vi "TSCANFD_SetData.vi"(8 "错误输入（无错误）":errorcluster, 10 "CANFD配置":T1={"硬件类型"=8, "硬件子类型"=0, "AArbRateKbps"=250.0, "AListenOnly"=enum."Normal", "Int120Ohm"=enum."Enable", "EnableChannel"=enum."Enable", "AHwChannel"=0, "AAppChannel"=0, "ADataRateKbps"=250.0, "AControllerType"=0, "AControllerMode"=0} {"硬件类型" items=["BUS_UNKNOWN_TYPE", "TS_TCP_DEVICE", "XL_USB_DEVICE", "TS_USB_DEVICE", "PEAK_USB_DEVICE", "KVASER_USB_DEVICE", "ZLG_USB_DEVICE", "ICS_USB_DEVICE", "TS_TC1005_DEVICE"]; "硬件子类型" items=["BUS_UNKNOWN_TYPE", "TSCAN_PRO_4", "TSCAN_LITE_2", "TSCANMini", "TSLinMini", "TSCANFDmini", "TSCAN_LIN_IO_2", "TSCAN_LITE_2", "TSCANLIN", "TSCAN_FD_Mini_1"]; "AHwChannel" items=["CHN1", "CHN2", "CHN3", "CHN4", "CHN5", "CHN6", "CHN7", "CHN8", "CHN9", "CHN10", "CHN11", "CHN12", "CHN13", "CHN14", "CHN15", "CHN16", "CHN17", "CHN18", "CHN19", "CHN20", "CHN21", "CHN22", "CHN23", "CHN24", "CHN25", "CHN26", "CHN27", "CHN28", "CHN29", "CHN30", "CHN31", "CHN32"]; "AAppChannel" items=["CHN1", "CHN2", "CHN3", "CHN4", "CHN5", "CHN6", "CHN7", "CHN8", "CHN9", "CHN10", "CHN11", "CHN12", "CHN13", "CHN14", "CHN15", "CHN16", "CHN17", "CHN18", "CHN19", "CHN20", "CHN21", "CHN22", "CHN23", "CHN24", "CHN25", "CHN26", "CHN27", "CHN28", "CHN29", "CHN30", "CHN31", "CHN32"]; "AControllerType" items=["lfdtCAN", "lfdtISOFDCAN", "lfdtNonISOFDFDCAN"]; "AControllerMode" items=["lfdmNormal", "lfdmACKOff", "lfdmRestricted"]}, 11 "路径输入":path) -> (0 "错误输出":errorcluster, 2 "AAPPChannel":i32, 3 "路径输出":path, 4 "Set_Baudrated_Successfully":bool, 6 "Mapping_Successfully":bool)   [LabVIEW 2019]
panel:
  # "用N路can通道，设置N路CAN通道"
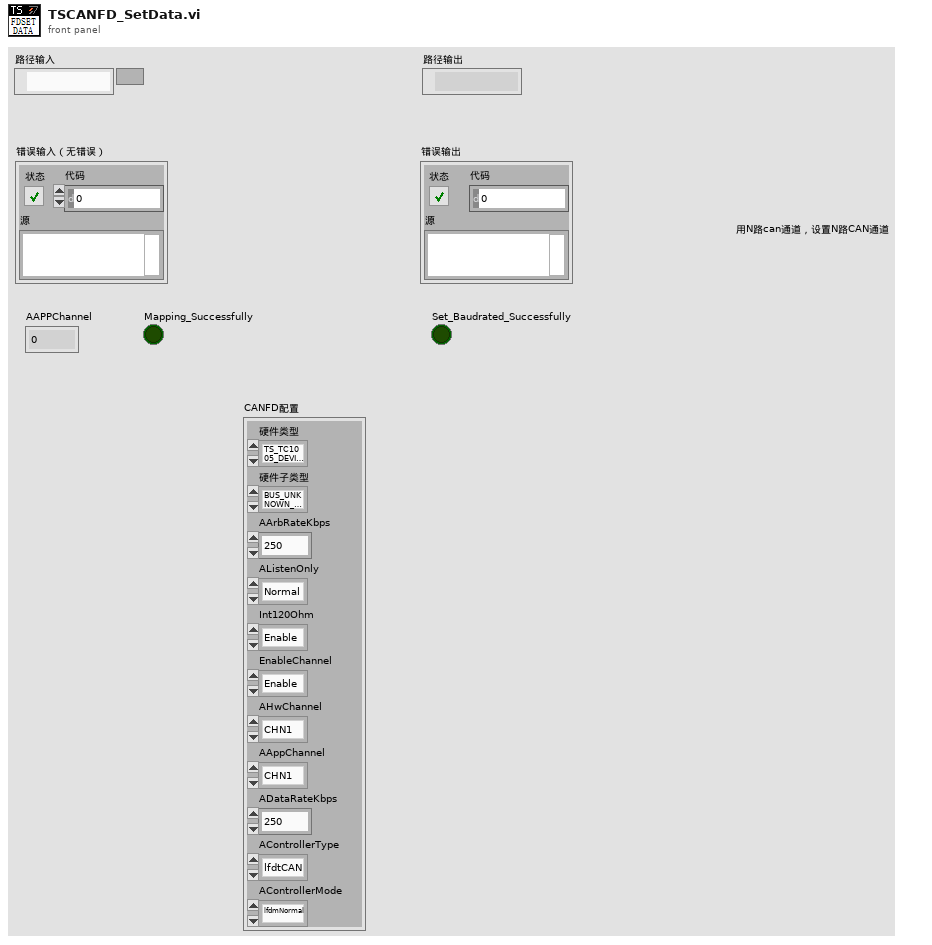
[diagram p1: front panel]
types:
  T1 = cluster{"硬件类型":i32, "硬件子类型":i32, "AArbRateKbps":sgl, "AListenOnly":enum16{"Normal", "ListenOnly"}, "Int120Ohm":enum16{"Disable", "Enable"}, "EnableChannel":enum16{"Disable", "Enable"}, "AHwChannel":i32, "AAppChannel":i32, "ADataRateKbps":sgl, "AControllerType":i32, "AControllerMode":i32}
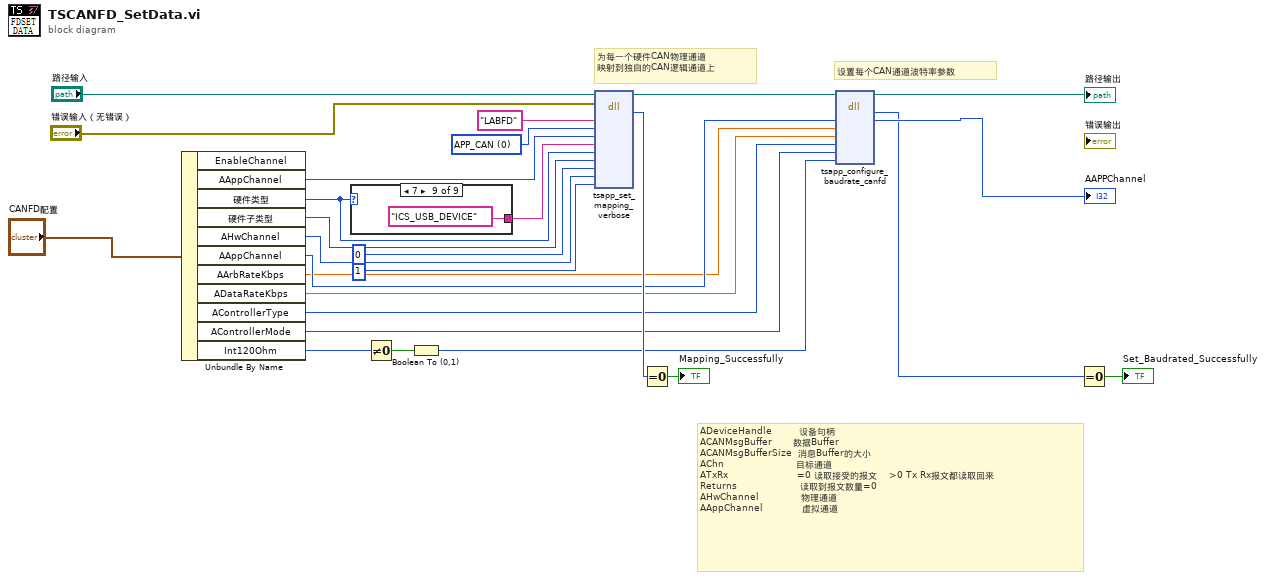
[diagram p0: block diagram]
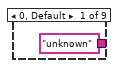
[diagram p2: hidden frame]
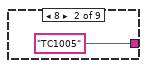
[diagram p3: hidden frame]
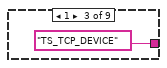
[diagram p4: hidden frame]
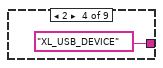
[diagram p5: hidden frame]
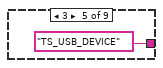
[diagram p6: hidden frame]
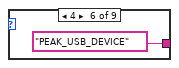
[diagram p7: hidden frame]
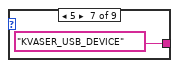
[diagram p8: hidden frame]
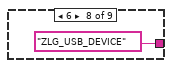
[diagram p9: hidden frame]
diagram:
  w26 = 0 items=["APP_CAN", "APP_LIN"] ("AAppChannelType")
  # "ADeviceHandle         设备句柄\nACANMsgBuffer       数据Buffer\nACANMsgBufferSize  消息Buffer的大小\nAChn                        目标通道\nATxRx                       =0 读取接受的报文    >0 Tx Rx报文都读取回来\nReturns                     读取到报文数量=0\nAHwChannel              物理通道\nAAppChannel             虚拟通道"
  # "设置每个CAN通道波特率参数"
  # "为每一个硬件CAN物理通道\n映射到独自的CAN逻辑通道上"
  n1 = Unbundle By Name("CANFD配置") -> ("AAppChannel"=w25:i32, "硬件类型"=w23:i32, "硬件子类型"=w22:i32, "AHwChannel"=w20:i32, "AAppChannel"=w9:i32, "AArbRateKbps"=w7:sgl, "ADataRateKbps"=w6:sgl, "AControllerType"=w5:i32, "AControllerMode"=w4:i32, "Int120Ohm"=w17:enum16{"Disable", "Enable"})  [unwired: 1 out]
  n2 = case shown="7" w23 {
    tunnel: ["unknown" ("AHardwareName") "TC1005" ("AHardwareName") "TS_TCP_DEVICE" ("AHardwareName") "XL_USB_DEVICE" ("AHardwareName") "TS_USB_DEVICE" ("AHardwareName") "PEAK_USB_DEVICE" ("AHardwareName") "KVASER_USB_DEVICE" ("AHardwareName") "ZLG_USB_DEVICE" ("AHardwareName") "ICS_USB_DEVICE" ("AHardwareName")] -> w24
    frame 0, Default {
    }
    frame 8 {
    }
    frame 1 {
    }
    frame 2 {
    }
    frame 3 {
    }
    frame 4 {
    }
    frame 5 {
    }
    frame 6 {
    }
    frame 7 {
    }
  }
  n3 = Not Equal To 0?(x=w17) -> (x != 0?=w18:bool)
  n4 = Boolean To (0,1)(Boolean=w18) -> (0, 1=w8:i16)
  n5 = dll-call lib="PTH2Habs CUsers\nAdministratorDesktopTS_Can通讯PathTSMaster.dll" fn="tsapp_set_mapping_verbose"(path in="路径输入", error in="错误输入（无错误）", "FAPppName"="LABFD" ("AppName"), "AChnType"=w26, "FAppChannelIndex"=w25, "AHWDeviceName"=w24, "AHWDeviceType"=w23, "AHWDeviceSubType"=w22, "AldHW"=0, "AldHWChn"=w20, "FMappingDisabled"=u32 1) -> (path out=w10:path, "tsapp_set_mapping_verbose"=w14:i32)  [unwired: 10 in, 1 out]
  n6 = Equal To 0?(x=w14) -> (x = 0?=→"Mapping_Successfully":bool)
  n7 = dll-call lib="PTH27abs EDemo同星\nTSCAN_V1.0ConfigTSMaster.dll" fn="tsapp_configure_baudrate_canfd"(path in=w10, "ALdxChn"=w9, "AArbRateKbps"=w7, "ADataRateKbps"=w6, "AControllerType"=w5, "AControllerMode"=w4, "AlnstallTermResistor120Ohm"=w8) -> (path out=→"路径输出":path, "tsapp_configure_baudrate_can"=w1:i32, "ALdxChn"=→"AAPPChannel":i32)  [unwired: 7 in, 1 out]
  n8 = Equal To 0?(x=w1) -> (x = 0?=→"Set_Baudrated_Successfully":bool)
